vi "Main On Save Action VI.vi"(8 "error in (no error)":errorcluster, 11 "Device Item Ref in":T1 format="%.0x") -> (0 "error out":errorcluster, 3 "Device Item Ref out":T1 format="%.0x")   [LabVIEW 2019, in "Ballard Arinc-429 System Explorer.lvlib"]
uses:
  Ballard Arinc-429 System Explorer.lvlib
  <vilib>/NI VeriStand/Custom Device API/Custom Device Item Ref.ctl
  Shared/Controls and Global/Global.vi
  <vilib>/NI VeriStand/Custom Device Tools/Custom Device Utility Library/NI VeriStand - Search for All Items by GUID.vi
  <vilib>/NI VeriStand/Custom Device API/Get Item Property (I32).vi
  <vilib>/NI VeriStand/Custom Device API/Get Item Property (Double).vi
  <userlib>/_OpenG.lib/array/array.llb/Remove Duplicates from 1D Array (U64)__ogtk.vi
  <vilib>/NI VeriStand/Custom Device API/Set Item Property (Double).vi
  <vilib>/NI VeriStand/Custom Device API/Custom Device API.lvlib
  <vilib>/NI VeriStand/Custom Device Tools/Custom Device Utility Library/Custom Device Utility Library.lvlib
  Shared/Ballard Arinc-429 Shared.lvlib
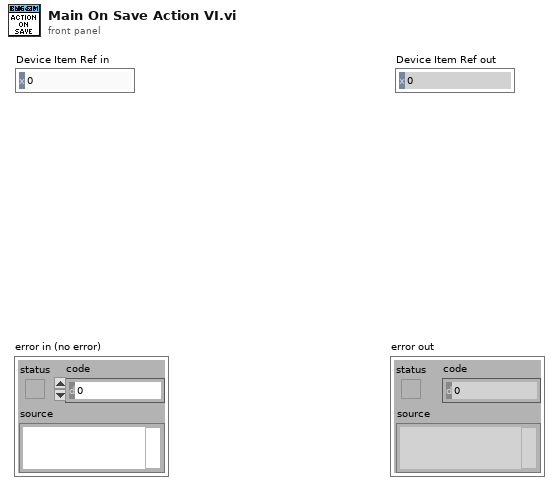
[diagram p1: front panel]
types:
  T1 = typedef "Custom Device API.lvlib/Custom Device Item Ref.ctl" = u64
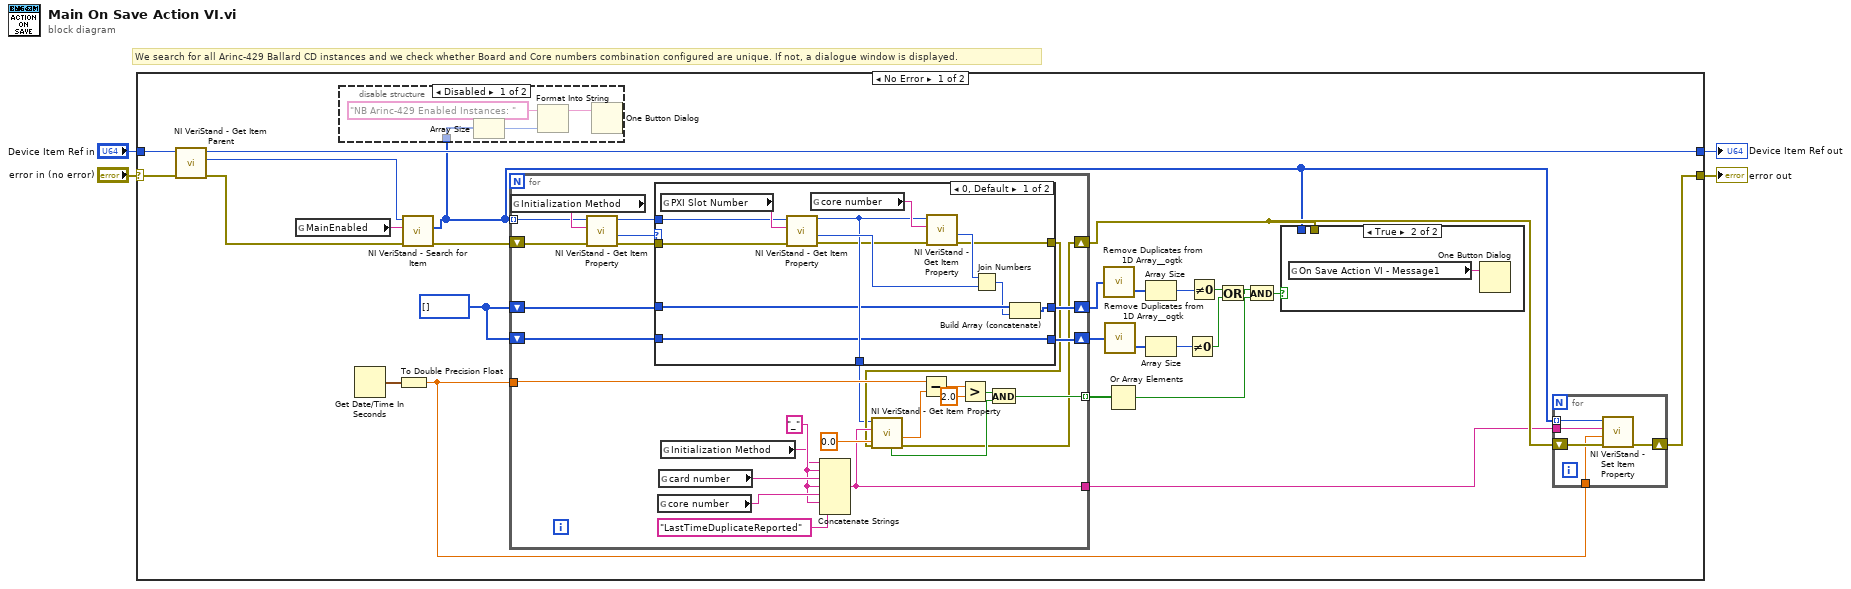
[diagram p0: block diagram]
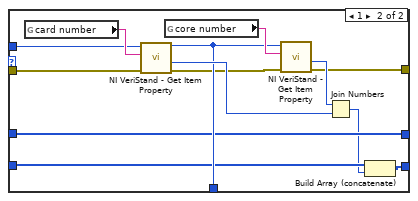
[diagram p4: hidden frame]
diagram:
  # "We search for all Arinc-429 Ballard CD instances and we check whether Board and Core numbers combination configured are unique. If not, a dialogue window is displayed."
  n1 = case shown="No Error" "error in (no error)" {
    selector: "error in (no error)" -> [w30 w95]
    tunnel: [w13 w95] -> w3
    tunnel: "Device Item Ref in" -> [w29 w94]
    tunnel: [w28 w94] -> w1
    frame No Error {
      w12 = u64[] []
      n2 = call <vilib>:"NI VeriStand - Get Item Parent.vi"("error in (no error)"=w30, "Item Ref in"=w29) -> ("error out"=w26:errorcluster, "Parent Ref"=w27:T1, "Item Ref out"=w28:T1)  [unwired: 6 in, 1 out]
      n3 = global read "Global.vi" "MainEnabled"() -> (w25:string)
      n4 = Get Date/Time In Seconds() -> (seconds since 1Jan1904=w21:timestamp)
      n5 = To Double Precision Float(number=w21) -> (double precision float=w18:dbl)
      n6 = call-poly <vilib>:"NI VeriStand - Search for Item.vi"("error in"=w26, "Item GUID"=w25, "Section Ref in"=w27) -> ("error out"=w24:errorcluster, "Item Refs"=w20:T1[])  [unwired: 5 in, 2 out]
      n7 = disable-structure shown="Disabled" {
        disable-tunnel: w20 -> [w39 _]
        frame Disabled {
          n8 = Array Size(array=w39) -> (size(s)=w38:i32)
          n9 = Format Into String(initial string="NB Arinc-429 Enabled Instances: ", w38) -> (resulting string=w37:string)  [unwired: 2 in, 1 out]
          n10 = One Button Dialog(message=w37) -> ()  [unwired: 1 in, 1 out]
        }
        frame Enabled {
        }
      }
      n11 = for {
        tunnel: w20 -> [w54] mode=indexing
        shift-right: [w42] -> w22
        shift-left: w24 -> [w52]
        tunnel: w18 -> [w65]
        tunnel: [w59] -> w15 mode=indexing
        tunnel: [w58] -> w19
        shift-right: [w48] -> w11
        shift-left: w12 -> [w49]
        shift-right: [w46] -> w10
        shift-left: w12 -> [w47]
        w45 = "_"
        n12 = global read "Global.vi" "Initialization Method"() -> (w55:string)
        n13 = call-poly <vilib>:"NI VeriStand - Get Item Property.vi"("error in (no error)"=w52, "Property Name"=w55, "Item Ref in"=w54) -> ("error out"=w51:errorcluster, "Value"=w50:i32, "Item Ref out"=w53:T1)  [unwired: 5 in, 1 out]
        n14 = case shown="0, Default" w50 {
          tunnel: [w76 w89] -> w43
          tunnel: [w75 w88] -> w41
          tunnel: w53 -> [w74 w87]
          tunnel: w51 -> [w73 w86]
          tunnel: w49 -> [w72 w85]
          tunnel: [w71 w85] -> w48
          tunnel: w47 -> [w70 w84]
          tunnel: [w70 w83] -> w46
          frame 0, Default {
            n15 = global read "Global.vi" "PXI Slot Number"() -> (w80:string)
            n16 = call-poly <vilib>:"NI VeriStand - Get Item Property.vi"("error in (no error)"=w73, "Property Name"=w80, "Item Ref in"=w74) -> ("error out"=w68:errorcluster, "Value"=w78:i32, "Item Ref out"=w75:T1)  [unwired: 5 in, 1 out]
            n17 = global read "Global.vi" "core number"() -> (w79:string)
            n18 = call-poly <vilib>:"NI VeriStand - Get Item Property.vi"("error in (no error)"=w68, "Property Name"=w79, "Item Ref in"=w75) -> ("error out"=w76:errorcluster, "Value"=w77:i32)  [unwired: 5 in, 2 out]
            n19 = Join Numbers(hi=w77, lo=w78) -> ((hi.lo)=w69:u64)
            n20 = Build Array (concatenate)(w72, w69) -> (w71:u64[])
          }
          frame 1 {
            n21 = global read "Global.vi" "card number"() -> (w93:string)
            n22 = call-poly <vilib>:"NI VeriStand - Get Item Property.vi"("error in (no error)"=w86, "Property Name"=w93, "Item Ref in"=w87) -> ("error out"=w81:errorcluster, "Value"=w91:i32, "Item Ref out"=w88:T1)  [unwired: 5 in, 1 out]
            n23 = global read "Global.vi" "core number"() -> (w92:string)
            n24 = call-poly <vilib>:"NI VeriStand - Get Item Property.vi"("error in (no error)"=w81, "Property Name"=w92, "Item Ref in"=w88) -> ("error out"=w89:errorcluster, "Value"=w90:i32)  [unwired: 5 in, 2 out]
            n25 = Join Numbers(hi=w90, lo=w91) -> ((hi.lo)=w82:u64)
            n26 = Build Array (concatenate)(w84, w82) -> (w83:u64[])
          }
        }
        n27 = global read "Global.vi" "core number"() -> (w57:string)
        n28 = global read "Global.vi" "card number"() -> (w67:string)
        n29 = global read "Global.vi" "Initialization Method"() -> (w44:string)
        n30 = Concatenate Strings(w44, w45, w67, w45, w57, w45, "LastTimeDuplicateReported") -> (w58:string)
        n31 = call-poly <vilib>:"NI VeriStand - Get Item Property.vi"("error in (no error)"=w43, "Default Value"=0.0, "Property Name"=w58, "Item Ref in"=w41) -> ("error out"=w42:errorcluster, "Value"=w64:dbl, "Found?"=w60:bool)  [unwired: 4 in, 1 out]
        n32 = Subtract(x=w65, y=w64) -> (x-y=w62:dbl)
        n33 = Greater?(x=w62, y=2.0) -> (0:w61:bool)
        n34 = And(x=w61, y=w60) -> (x .and. y?=w59:bool)
      }
      n35 = call-poly <userlib>:"Remove Duplicates from 1D Array__ogtk.vi"("Input Array"=w11) -> ("indices of removed elements"=w23:i32[])  [unwired: 1 out]
      n36 = call-poly <userlib>:"Remove Duplicates from 1D Array__ogtk.vi"("Input Array"=w10) -> ("indices of removed elements"=w9:i32[])  [unwired: 1 out]
      n37 = Or Array Elements(Boolean array=w15) -> (logical OR=w14:bool)
      n38 = Array Size(array=w23) -> (size(s)=w16:i32)
      n39 = Array Size(array=w9) -> (size(s)=w8:i32)
      n40 = Not Equal To 0?(x=w8) -> (x != 0?=w6:bool)
      n41 = Not Equal To 0?(x=w16) -> (x != 0?=w7:bool)
      n42 = Or(x=w7, y=w6) -> (x .or. y?=w5:bool)
      n43 = And(x=w5, y=w14) -> (x .and. y?=w17:bool)
      n44 = case shown="True" w17 {
        tunnel: w22 -> [_ _]
        tunnel: w20 -> [_ _]
        frame False {
        }
        frame True {
          n45 = global read "Global.vi" "On Save Action VI - Message1"() -> (w40:string)
          n46 = One Button Dialog(message=w40) -> ()  [unwired: 1 in, 1 out]
        }
      }
      n47 = for {
        shift-right: [w34] -> w13
        shift-left: w22 -> [w35]
        tunnel: w20 -> [w33] mode=indexing
        tunnel: w19 -> [w32]
        tunnel: w18 -> [w31]
        n48 = call-poly <vilib>:"NI VeriStand - Set Item Property.vi"("error in (no error)"=w35, "Value"=w31, "Property Name"=w32, "Item Ref in"=w33) -> ("error out"=w34:errorcluster)  [unwired: 5 in, 2 out]
      }
    }
    frame Error {
    }
  }
  "error out" <- w3
  "Device Item Ref out" <- w1
